vi "Get System Channels.vi"(8 "error in (no error)":errorcluster, 11 "target in":refnum<k39>) -> (0 "error out":errorcluster, 1 "channels":T1[](array[typedef]) format="%.0x", 2 "names":string[](array[string]), 3 "target out":refnum<k39>)   [LabVIEW 2027, in "Embedded Data Logger Scripting Unit Tests.lvclass"]
uses:
  Embedded Data Logger Scripting Unit Tests.lvclass
  Embedded Data Logger Scripting Unit Tests.lvclass/Embedded Data Logger Scripting Unit Tests.ctl
  C:/NetCore/niveristand-embedded-data-logger-custom-device/Source/Scripting/Tests/Unit/Get System Channels.vi/NationalInstruments.VeriStand.SystemDefinitionAPI
  NationalInstruments.VeriStand.SystemDefinitionAPI
  C:/NetCoreDLL/NationalInstruments.VeriStand.SystemDefinitionAPI.dll
  NetCoreDLL/NationalInstruments.VeriStand.SystemDefinitionAPI.dll
  <vilib>/NI VeriStand/Custom Device API/Custom Device Item Ref.ctl
  <vilib>/NI VeriStand/Custom Device API/Custom Device API.lvlib
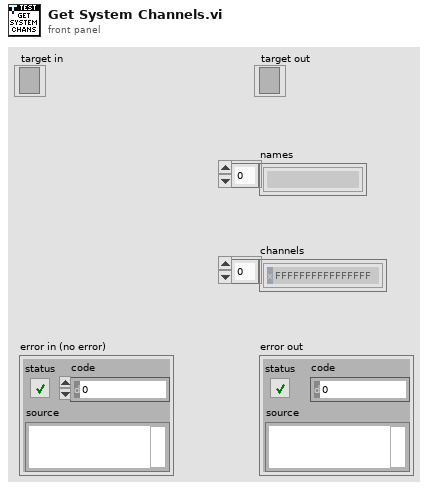
[diagram p1: front panel]
types:
  T1 = typedef "Custom Device API.lvlib/Custom Device Item Ref.ctl" = u64
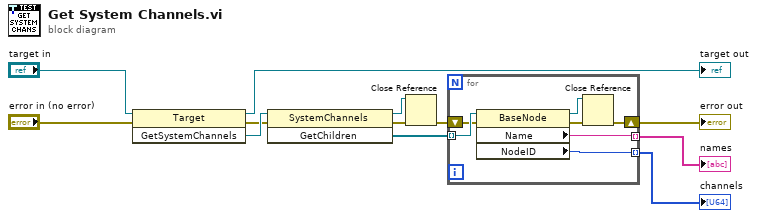
[diagram p0: block diagram]
diagram:
  n1 = invoke class="Target" method="GetSystemChannels"(reference="target in", error in="error in (no error)") -> (reference out=→"target out":refnum<k39>, error out=w5:errorcluster, "GetSystemChannels"=w9:refnum<k39>)  [unwired: 1 in]
  n2 = invoke class="SystemChannels" method="GetChildren"(reference=w9, error in=w5) -> (reference out=w2:refnum<k39>, error out=w4:errorcluster, "GetChildren"=w10:refnum<k39>[])  [unwired: 1 in]
  n3 = Close Reference(reference=w2, error in (no error)=w4) -> (error out=w3:errorcluster)
  n4 = for {
    tunnel: w10 -> [w19] mode=indexing
    tunnel: [w14] -> w7 mode=indexing
    shift-right: [w16] -> w12
    shift-left: w3 -> [w17]
    tunnel: [w13] -> w1 mode=indexing
    n5 = property class="BaseNode"(reference=w19, error in=w17) -> (reference out=w15:refnum<k39>, error out=w18:errorcluster, "Name"=w13:string, "NodeID"=w14:u64)
    n6 = Close Reference(reference=w15, error in (no error)=w18) -> (error out=w16:errorcluster)
  }
  "error out" <- w12
  "channels" <- w7
  "names" <- w1
